vi "2023_day21_Task1.vi"() -> ()   [LabVIEW 2021]
uses:
  a007553b-196c-4698-b023-200d8bc566d7.vi
  <userlib>/_OpenG.lib/array/array.llb/Index 2D Array Elements (String)__ogtk.vi
  <userlib>/_OpenG.lib/array/array.llb/Search 1D Array (Boolean)__ogtk.vi
  <userlib>/_OpenG.lib/array/array.llb/Delete Elements from 2D Array (I32)__ogtk.vi
panel:
  out "Task 1":i32
  in  "Switch":bool caption="Ex. Data  vs.  User Data"
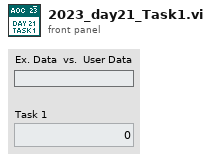
[diagram p1: front panel]
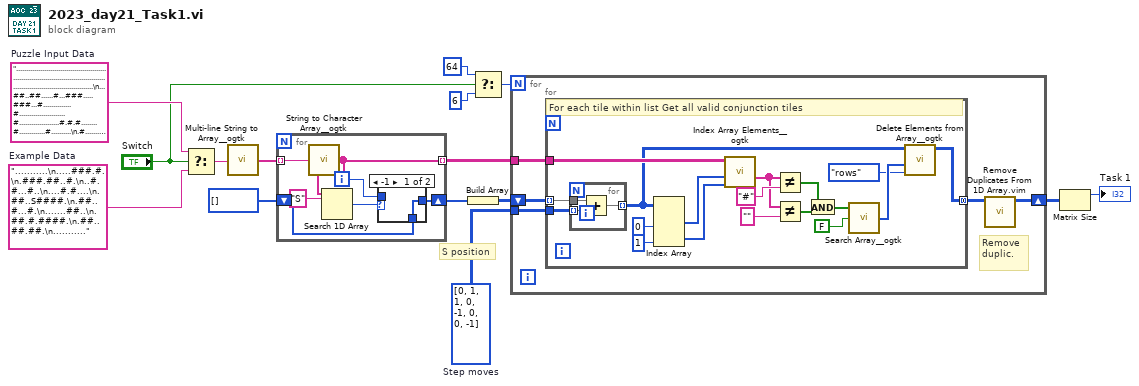
[diagram p0: block diagram]
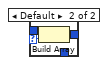
[diagram p2: hidden frame]
diagram:
  w7 = i32[][] [[0, 1], [1, 0], [-1, 0], [0, -1]]  # Step moves
  w14 = "...................................................................................................................................\n...##..##......#...###.....###...#..............#.......................#....................#.#.#........#.............#..........\n.#..........#...#.#..#....#.#........#.....#..#...........#..................................#.....#.............#..#.#.#.....##...\n..#....#...................#..........#....#..........#.#..........................#.............#.#.#..............#.#............\n....#...#............#....#.#.#..#.........#..#......#..#....................#..#.#.............##............#.............##.....\n..........#............##..#....#.#.............................#.................#....##.##.##....#...##..#.....#.....#.....#.....\n......#..#...#.#..............#.#......#.#.......#....#........##..#.......#.#.#.....#......#..#.#..#.......#.........##...........\n...#..#..............#....#.#.......#......#....#.....#.............#........................#.......#..#........#..........##.....\n...#....#...#..#..#.....#..#....#.#...#.....#...................#.............#...#.....#..#..#..#.........#.....#.......#.........\n....#....#.......##..........#............#..#.......................................#.#......#.#...#.....#...#........#...#.......\n.....#...###....#....#...#..............#.........................#.##......................##..#..#.#.##.........#...#............\n...........#.......#.......#.....#...............#................#.#..##...........##..#.......###.#.#..#...#.#..........#........\n..#......###..........#.#.......#..#..#..##....#...................#....#........###..#.#.....#...........#..............#..#....#.\n....#.........#.#....#.........#..#.#.....#...#.........#..#........#...................#....#.#....#..#.#.....#....#...##..#.##...\n....#..#....#.............#.......#.#...#..............#..........#....#...#........##...#.......#.........#.##............##......\n.......#.#...........#....#...................................#....#........#...........#.#.###...#.........#.##.#....#...#.#..##..\n....#..#........#..#..#.#..#.........#......#.............#..............#..................#.....#.#.....#..#.........#...#.......\n........##...##..#......##...........#.................#.....###..#....#...#..........#.#..............#..#......................#.\n.#............#.......##...........#.....................#.........#.........................##.....#..###.....#...#..###........#.\n...........##...#............#......#.................#.....#..#...#...#.......#.........#..##.........#....###.....#.#......##..#.\n.#....##.......#.......#...#..##..#.#...#............#.#...#......#...........................#.........#........#.........##......\n..#...#...##.#.......................##...........#..#........#.#.....##..#.##.#..#.......#..#.....#.####.#.......#......#.........\n.....#.##.#...##.#...........#.................#.....#....#.#..#.......#.........................#.#......#.##..#....#.#........#..\n.....##.###..#...................#.........................#..#....#..#....................................#..##..#.#...#..#..#.#..\n.#......#.#......#.............#.##..#.........##...##..........#.........#..#...#.#...........#.....##.......#.............##.#...\n....#..........#.#....#...#.#....................#.###.........#......##...#.........#............#........#....#..#....##.#...##..\n.............##.....#...#...#......#.............#............##.....#.......#.#........................#..#..........#...#........\n..#......##............#...#.........................##..##..............#..#......#.................##........#...............##..\n..#.......#...#......#...................#........#..#...##............##..#.....#..........................#.#..........#.........\n...##..#...##..........##....###.........#.......##..................#.......#....................#...........#.#........#.........\n......#....#......#.......#...#....................#..#........#..#......#..#.#....##.........................#.#....#.#....#....#.\n.....#......................#................#......##......##.#.........#..##.........#...............##.......#.........#........\n.#.#......#.#....#..#...#..............#......#..#.#.....#..........##.....#..#........#...#.#.........#..#.....................#..\n...#.##.#..#..#...#.#................###....................##.....#.#....#.........#......#..#..........##.#....#......#..#.......\n...#.................#.............#................#.................###..............#.................#..#......#.....#......##.\n.#.#.....#..#..........#...........#.#............#.##..#......#..##....#.#..###.......##.#.....#.........##...#.#...........#.....\n..#...#................#....................#..#..........#...............#.....#..#..####................#...............#........\n..........#..........#..............#........#...##...............#.....#...#...#..##.....#...#...........##.#.....##.#......#.....\n....#......#.......#...#.......#........#....#.....#..............#....#..##..#......#........#...............#.................#..\n.#.............#...............#...............#..#...#..#.#...#..#.......#....................#....#........#..##........#........\n.....................................#....###....#...#.....##.#.......#.........#.#.....#........#...........#...........##......#.\n.......#.##...#..............#..##..#...#...........#.##..##..#....#..#.........#........#.#.....................#.......#.......#.\n..#......##...................#..........#........##.....#..........#...#.#....#.#....#............##..............#...#.#.#.......\n...#.#.##.#.#.......................##......#.......#.........#.........#..........#........#.#.....#.#.............#.........#....\n.#.#...........#..................#....#......#.#............#....#.#..#...#..#..##.#............................#.#........#.##...\n..#...#....#...................#....#..........#.......................#.....##..#...#.#.#.......#...#..#.........#......##........\n.......#.................#...#........#....#.................#......................#...#.........##..................#......#.....\n..#..#....#..#...............#................#..#.#.....#.#..#.........###.......................#.#..#....#..........#...........\n......#...#..#...........#......................#..#............................#.....#........#.....##...#............#...........\n...........................##..#....#....#.....#....#....#...#........#.......#.........#.#..........##...#..................#..#..\n......#.....................#.....#.......#.#.....#.............#....#...#......#....#..#..........#........#...........#..........\n..#...#.............#..............#.#....#....#.....#....#...#.#......#.....#.#...........#.#.........#.#..................#..###.\n..#..............#....##......#.##..................#...##.........#..........#.................#..........#...................#...\n................#.##...#......##.........#.#...#..####.#.............#...#....#.........#.................................#........\n....#..........................#.......#...............#......#.......#...###.##.....#.#.#....#..###....#...#...##...........##....\n...#.#...............#..................#.........#...#.#..............#.....#.......#...#.##...#..#.......#.....#...........#.....\n.....#.....................#.#.#.....#.#.....#..#..##...#.....#...........#...##........#..#.......#.#...#....#..#............#....\n..#..........#....##..#.....###.#...............................#.#.##.#...#....##........#...#.....#....#............#.......#....\n.#...........#...#..#.....#..........#............#.......##......#.................#.#...#..##........#...............#...........\n.#................#........##.#.#.....#.#.............#.....#..#..##...............#..#................#.......#...#...##.......##.\n.#........#.##........##..#.#.##.....#..###..#......##...#......#..........#...............#.....#....#......#.....................\n............#.........#..............#.....#..#......................#...#.##.##...###..#..........###........###..................\n...........#...##.............#......#.....#.#...#...#.#..#....#..#............#....#..#.....#.#.........#.....#..#.###....#.......\n.........#........#.......#..#..##..#........#.#.#...........#....................##..#....#..#.....##.......##...##...............\n.......#....##..........##.....#...##....#.........#..#...................#......###.....#........#.....................#.#.#......\n.................................................................S.................................................................\n.....#...........#...#....#...#..#.........#.......##.#.............................#...#....#......#......#...#.#......#....#.....\n........###...#.......................#...........#.....#.#.........#.#......#...#.....#..#...###.....#.#....#..........#..........\n...............#.#............#.#......#...#..#.......#..#.#..#....##.#..#....#...............#.##.#..#...#...#..#.................\n.............#.##..........#........#.#........###.....#..............#.......#..........##...........#........#...#...............\n...........#.#.#........#......###.....#.#......#.#..##..#..#...#...##.#.#...##.......#........#..#.#.##...###...........#.........\n..........##..............#......#.............#..#.#....#..#.....#.#...#..........##............#...#.##.....#.#..#...............\n.#.#...............#.#............##.......#...#..#....#.....#........#.#..###...#.....#.........#................#..#.............\n.............#...#........#....#....#..........##.#....#......#.....#.........#..#........#.......###....#.#....#....##............\n...#............#.#......#...#....#..............#.....#..##....#.....#....#.....#...#...#.#..#.........#.#.........#..............\n..............#.......#...........#..............#.#.......#..#.#......#...##.......#................#...#.....#...#...............\n...##...........................#...#...#.......#............#.#.....#...#....#..#......#..#.##....#.#...#...#.................#.#.\n...#....#...........#.........##...#............#...............#...................................##..#......#..#..............#.\n...##.#.#.............#....#.##.#........#.....#.#...#.....##...........#.....................#...#..#......#............##.....#..\n...#..#...#...............#.#......#....#.#.#......#...................#......#.....##....#....#....##...#......#..............#...\n......#..#.........#.................#...#................#.........#..................................................#....#......\n.#..........#..........#..................#.#...#....#....#.#.........#..#...#........#......#.............#....................#..\n........#............#........#.......##......##....#................#.......#....#.#.....#............#.#.#...............###.....\n.##........#..........#...#......##..#.##.#.....##.........................#.....##.#...#......#.#......#..#..........#............\n....#....................#...#.......#...#.......#.....#......#...#..#...#......#.#..#...##.##..#.....##...........#..#.###........\n.#.....#........#..............#...#...#.........#.#................#.#.............##.#....#..#.....................#.....#..###..\n......#...#.#..#.............##.#........#.....................#........#....#...........#....##......................#............\n..#.....##...#..#.#.........#.#.......#.#..#......#..........#.##....#..#..................#.........#..#........#....##...........\n..#...#.#....#.#...................##......##...........#...#.............#..........#.##..#.#......#..................#..#.#...##.\n...##...#........#.#.........#...#.....#.#...##...#...#..#.#.........#.....#..#....#.###...#........#.............#.........#....#.\n.........#...#.#...#.#.................#............#........................#.#.....#.........#................#.....#..#......#..\n...........#.#..#.............##........#..........#....#...........#....#.....#....#....#.#......##.........#..##....#..##........\n.........#..................................#..#...............#...#..#...#...#..#......#.#..#.............#...........#.#..#...##.\n.#.#......#..#.......#.##........#......#....#................#...#...##..##....#.....#..........#.........#....#..#.#.........#...\n.....#.....#.........#............#....#.....................#....#.##...#......................#................#.#.#...#.........\n.....#.............##..#..........#..#..............##..#.................##........###.....#.#.........#.#.#...............#......\n.#.#.#...#.#..............#...............#...............#..#.....#......#..............................#.......#.#...#.#...#.....\n.................#........#...............#.........................................#......................#....#............#...#.\n.#...#.###...........#...#..##...............#.........#...##....................#...........#...............#....##...........#.#.\n..###...#.#.........##.................#.#.....#..##...........#....##........#...#...................##..##...#................#..\n...#.................#.....#...........#....#...##...#.......#............#.....#.#........#........#...#...##...#.##..............\n.......#....#.........#.#.....#.#.......#.....#....#...#.............#.....#.....#.##.....................#.###...........#........\n................#....#..#.......#.............#......#.......#.................#.#................#..........#.....##...#..#....#..\n........#...#...#.#......##......#.........#.......................#.........#...#.....................#..........#.#..#...#.......\n....#.......##......##....##.................#.....#.#.#....#...#...........#.......................#........#....#....#.....#...#.\n.#..##..##.........#......#.........#.......#....#....#...#.....#..#.....#.#............................#...#..................#.#.\n...#......#............##.....##.............##.................#..#....#.#...#....#......................##....#.....#........#...\n........#....#....#..........#.###....#................#..##......#..#...#..#......#..........##...............#..#.........#...#..\n.....#...#.##.....#....#.##.........#............##....#..#.#.....#.............#...................#..#............#..#..#.#....#.\n.....#..#.........##..#...........#....#............#.#...........#..............##.......#.#...........#..####.....##.#.##........\n...#.#.#.##.#.#..#.....#........###..#............#........##......##.#..........................####........##.#.....#......#.....\n.##.#.#...##..#........##....#........#............#...#...#......#....#....##..#...........#.#.........#.##...#...#...#...#.#.....\n......#.#..#.#........##.#....#.#...#.###..#...........#...................#.................#.#.#............##.#...#.#.........#.\n........#.#....#...#...#..........#.#..#..#...........#..#...#.....##......#.....................##..#........#.....#.#.....#....#.\n..#.......##....##............##...............................#......#.#..#.............#..........................#....#.........\n.......#....#................#...........#...##................#...#.#....#...............#....##.......................#.#.....#..\n..........#...........#..#..#.....#...........##...........#......#.#.#.#..........#..........#.....#......................###.....\n....#.......##...........#..........#..###.#.........................#....#..........#.#.........#......#............#..#.....#..#.\n...#.#...#...#.............#.......#...#.##..............................#........##.......##..#...#......................#........\n...........##.............#....##....#.#...#.#..............#..#..................#.......#......#.......#.................#..#....\n.#.##..#......#...#..#........#.......#.#.#....#...............#........................#..........#...............................\n........#...........#....#...#...##..#.#....###................#...#.................#..................#.......#....#........#..#.\n.........#.###.#....#..#..##..........#.#.......#............................#..##....#.....#....#....#.#...##......##.............\n..#.#..##.#........#..#.#...#........#...#...#.....................##...........#.....#...#.#.#...#.......#..#..#.........#..#..#..\n.....#..........####....##..##......#.............#...#...........#........#..........#.............###...#.#.#...#................\n..#.....#...#....#.#.........#....#..#.......##.....#.............#........#............#...###.........#...#......................\n.##..............#..#....#..#......#....##..#......#.###.#..................#...............#.#..#..#.##..........#............#.#.\n..#..#..#.....................#.#..............##...#.....#....................#..##...#.........#...........#..##.........#....#..\n....#...............#.......#.#....##....#..#..........................#.......#.##...........#.......#....#.#........#..#.........\n.....##.......#.................................#........#..................#..#.#......#....#..#....#...#.........................\n..................................................................................................................................."  # Puzzle Input Data
  w15 = "...........\n.....###.#.\n.###.##..#.\n..#.#...#..\n....#.#....\n.##..S####.\n.##..#...#.\n.......##..\n.##.#.####.\n.##..##.##.\n..........."  # Example Data
  # "S position"
  n1 = Select(t=w14, s="Switch", f=w15) -> (s? t:f=w13:string)
  n2 = call <userlib>:"Multi-line String to Array__ogtk.vi"("string"=w13) -> ("lines"=w12:string[])
  n3 = for {
    tunnel: w12 -> [w22] mode=indexing
    tunnel: [w21] -> w10 mode=indexing
    shift-right: [w17] -> w9
    shift-left: i32[] [] -> [w16]
    i -> [w18]
    n4 = call <userlib>:"String to Character Array__ogtk.vi"("Input String"=w22) -> ("Character Array"=w21:string[])
    n5 = Search 1D Array(1D array=w21, element="S") -> (index of element=w19:i32)  [unwired: 1 in]
    n6 = case shown="-1" w19 {
      selector: w19 -> [_ w26]
      tunnel: w18 -> [_ w25]
      tunnel: [w23 w24] -> w17
      tunnel: w16 -> [w23 _]
      frame -1 {
      }
      frame Default {
        n7 = Build Array(w25, w26) -> (w24:i32[])
      }
    }
  }
  n8 = Build Array(w9) -> (w8:i32[][])
  n9 = Select(t=64, s="Switch", f=6) -> (s? t:f=w2:i32)
  n10 = for {
    N: w2 -> [_]
    tunnel: w10 -> [w30]
    shift-right: [w27] -> w6
    shift-left: w8 -> [w29]
    tunnel: w7 -> [w31]
    # "Remove duplic."
    n11 = for {
      tunnel: w29 -> [w48] mode=indexing
      tunnel: w31 -> [w49]
      tunnel: w30 -> [w47]
      tunnel: [w32] -> w28 mode=concatenating
      # "For each tile within list Get all valid conjunction tiles"
      n12 = for {
        tunnel: w49 -> [w52] mode=indexing
        tunnel: w48 -> [w51]
        tunnel: [w50] -> w35 mode=indexing
        n13 = Add(x=w51, y=w52) -> (x+y=w50:i32[])
      }
      n14 = Index Array(array=w35, index (col) #1=0 ("index (row)"), index (col) #2=1 ("index (row)")) -> (element #1=w43:i32[], element #2=w42:i32[])  [unwired: 2 in]
      n15 = call-poly <userlib>:"Index Array Elements__ogtk.vi"("indices 1"=w42, "indices 0"=w43, "array"=w47) -> ("elements"=w45:string[])  [unwired: 8 in]
      n16 = Not Equal?(x=w45, y="#" ("element")) -> (x != y?=w39:bool[])
      n17 = Not Equal?(x=w45, y="" ("element")) -> (x != y?=w38:bool[])
      n18 = And(x=w39, y=w38) -> (x .and. y?=w37:bool[])
      n19 = call-poly <userlib>:"Search Array__ogtk.vi"("Array"=w37, "Element Data"=FALSE) -> ("Indices of Elements"=w34:i32[])  [unwired: 7 in]
      n20 = call-poly <userlib>:"Delete Elements from Array__ogtk.vi"("delete (rows or columns)"=enum16{"rows", "columns"}."rows", "indices"=w34, "array"=w35) -> ("array w/ subset deleted"=w32:i32[][])  [unwired: 7 in, 1 out]
    }
    n21 = call "Remove Duplicates From 1D Array.vim"("array"=w28) -> ("array with duplicates removed"=w27:i32[][])  [unwired: 10 in]
  }
  n22 = Matrix Size(0:w6) -> (1:→"Task 1":i32)  [unwired: 1 out]
